vi "Set BGK Color.vi"(8 "error in (no error)":errorcluster, 9 "color":u32(colorbox), 11 "XYGraph":refnum<vi>) -> (0 "error out":errorcluster, 3 "XYGraph out":refnum<vi>)   [LabVIEW 2019]
doc: "This sets the background color of a graph, but also the gridlines are automatically adjusted to offset from that color. It works by determining the luminance and adjusting the major and minor grids by a few percent up and down accordingly from that set color.\n\nThis allows graphs to be easily set with new BGK colors for display or printing or by the end user and still look good."
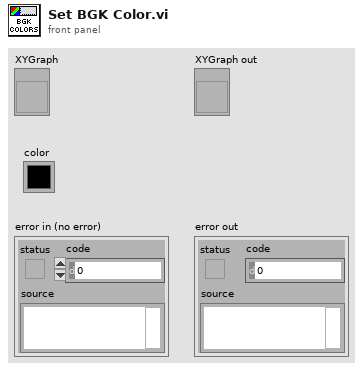
[diagram p1: front panel]
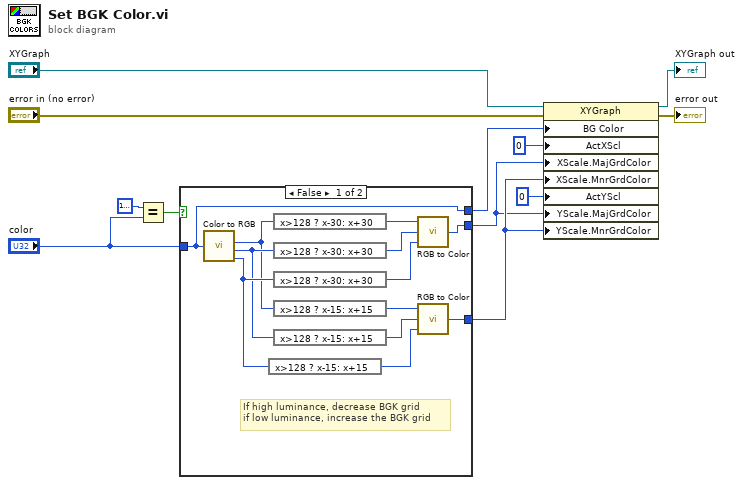
[diagram p0: block diagram]
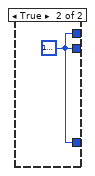
[diagram p2: hidden frame]
diagram:
  n1 = Equal?(x=u32 16777216, y="color") -> (x = y?=w3:bool)
  n2 = case shown="False" w3 {
    tunnel: [w24 w25] -> w11
    tunnel: [w23 w25] -> w10
    tunnel: "color" -> [w13 _]
    tunnel: [w13 w25] -> w4
    frame False {
      # "If high luminance, decrease BGK grid\nif low luminance, increase the BGK grid"
      n3 = call <vilib>:"Color to RGB.vi"("Color"=w13) -> ("R"=w14:u8, "G"=w15:u8, "B"=w16:u8)  [unwired: 1 out]
      n4 = expression code="x>128 ? x-15: x+15"(w16) -> (w22:u8)
      n5 = expression code="x>128 ? x-30: x+30"(w14) -> (w17:u8)
      n6 = expression code="x>128 ? x-30: x+30"(w15) -> (w18:u8)
      n7 = expression code="x>128 ? x-30: x+30"(w16) -> (w19:u8)
      n8 = expression code="x>128 ? x-15: x+15"(w14) -> (w20:u8)
      n9 = expression code="x>128 ? x-15: x+15"(w15) -> (w21:u8)
      n10 = call <vilib>:"RGB to Color.vi"("B"=w19, "G"=w18, "R"=w17) -> ("Color"=w23:u32)
      n11 = call <vilib>:"RGB to Color.vi"("B"=w22, "G"=w21, "R"=w20) -> ("Color"=w24:u32)
    }
    frame True {
      w25 = u32 16777216
    }
  }
  n12 = property class="XYGraph"(reference="XYGraph", error in="error in (no error)", "BG Color"=w4, "ActXScl"=0 ("Active X Scale"), "XScale.MajGrdColor"=w10, "XScale.MnrGrdColor"=w11, "ActYScl"=0 ("Active Y Scale"), "YScale.MajGrdColor"=w10, "YScale.MnrGrdColor"=w11) -> (reference out=→"XYGraph out":refnum<vi>, error out=→"error out":errorcluster)
